vi "Save XML Next to VI.vi"(5 "include size in file name? (F)":bool, 7 "layout keyword (\"\")":string, 8 "error in":errorcluster, 11 "VI refnum":refnum<vi>) -> (0 "error out":errorcluster, 1 "saved?":bool)   [LabVIEW 2010, in "NI_SE_Front Panel Layout.lvlib"]
uses:
  NI_SE_Front Panel Layout.lvlib
  VI Panel Layout/VI Panel Layout.lvclass
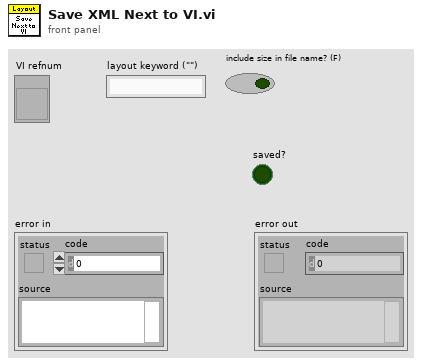
[diagram p1: front panel]
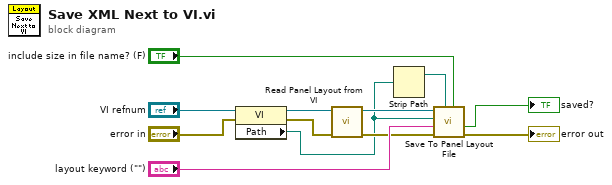
[diagram p0: block diagram]
diagram:
  n1 = property class="VI"(reference="VI refnum", error in="error in") -> (reference out=w6:refnum<vi>, error out=w3:errorcluster, "Path"=w2:path)
  n2 = call "Read Panel Layout from VI.vi"("error in"=w3, "VI refnum"=w6) -> ("error out"=w4:errorcluster, "panel layout out"=w5:refnum<class "VI Panel Layout.lvclass">)  [unwired: 8 in]
  n3 = Strip Path(path=w2) -> (stripped path=w1:path)  [unwired: 1 out]
  n4 = call "Save To Panel Layout File.vi"("include size in file name? (F)"="include size in file name? (F)", "panel layout folder (\"\")"=w1, "error in)"=w4, "layout keyword (\"\")"="layout keyword (\"\")", "VI path"=w2, "panel layout in"=w5) -> ("error out"=→"error out":errorcluster, "saved?"=→"saved?":bool)  [unwired: 3 in, 1 out]
